vi "Channel0_control.vi"(4 "V/DIV in":dbl, 6 "Boolean":bool, 7 "Measured amplitude":dbl, 9 "S/DIV in":dbl, 10 "Measured frequency":dbl, 11 "WaveformGraph in":refnum<vi>) -> (2 "V/DIV out":string, 3 "S/DIV out":string)   [LabVIEW 2019]
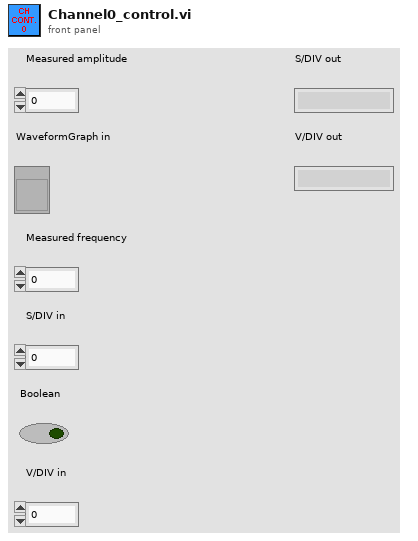
[diagram p1: front panel]
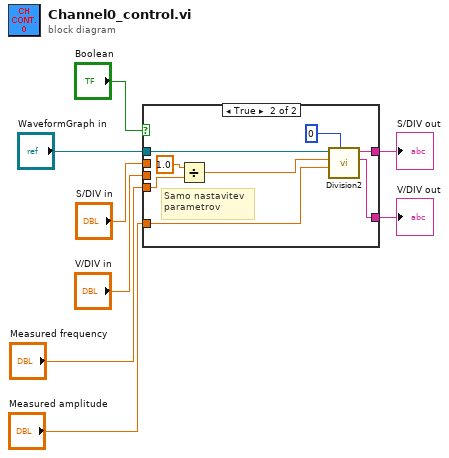
[diagram p0: block diagram]
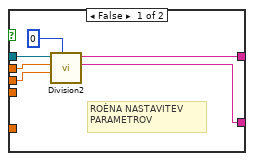
[diagram p2: hidden frame]
diagram:
  n1 = case shown="True" "Boolean" {
    tunnel: "S/DIV in" -> [w11 _]
    tunnel: [w14 w21] -> w2
    tunnel: [w13 w20] -> w3
    tunnel: "WaveformGraph in" -> [w12 w22]
    tunnel: "Measured frequency" -> [_ w16]
    tunnel: "Measured amplitude" -> [_ w17]
    tunnel: "V/DIV in" -> [w10 _]
    frame False {
      # "ROÈNA NASTAVITEV \nPARAMETROV"
      n2 = call "Division2.vi"("Scale_select"=u32 0, "V/div"=w10, "s/div"=w11, "WaveformGraph in"=w12) -> ("V/DIV"=w13:string, "S/DIV"=w14:string)  [unwired: 5 in, 1 out]
    }
    frame True {
      # "Samo nastavitev \nparametrov"
      n3 = Divide(x=1.0, y=w16) -> (x/y=w19:dbl)
      n4 = call "Division2.vi"("Scale_select"=u32 0, "V/div"=w17, "s/div"=w19, "WaveformGraph in"=w22) -> ("V/DIV"=w20:string, "S/DIV"=w21:string)  [unwired: 5 in, 1 out]
    }
  }
  "V/DIV out" <- w3
  "S/DIV out" <- w2
